vi "Example for Figure Window.vi"() -> ()   [LabVIEW 2020]
panel:
  out "Iteration number":i32
  in  "Stop":bool
  in  "new data":bool
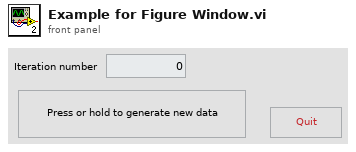
[diagram p1: front panel]
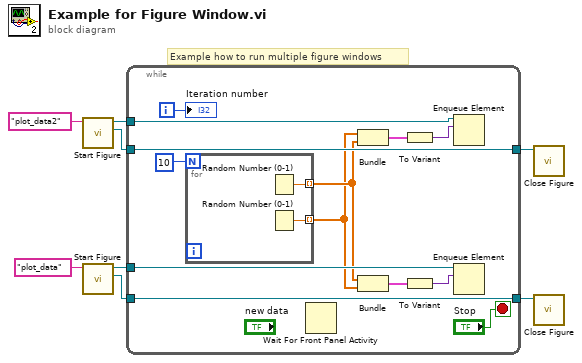
[diagram p0: block diagram]
diagram:
  # "Example how to run multiple figure windows"
  n1 = call "Start Figure.vi"("Qeue name (figure_data)"="plot_data2" ("name (unnamed)")) -> ("reference out"=w4:refnum<vi>, "queue out"=w5:refnum<queue>)  [unwired: 8 in, 1 out]
  n2 = call "Start Figure.vi"("Qeue name (figure_data)"="plot_data" ("name (unnamed)")) -> ("reference out"=w2:refnum<vi>, "queue out"=w6:refnum<queue>)  [unwired: 8 in, 1 out]
  n3 = while {
    tunnel: w6 -> [w20]
    tunnel: [w18] -> w1
    tunnel: w2 -> [w18]
    tunnel: [w17] -> w3
    tunnel: w4 -> [w17]
    tunnel: w5 -> [w16]
    i -> [w19]
    stop <- "Stop" stop-if-true
    n4 = for {
      N: 10 -> [_]
      tunnel: [w23] -> w11 mode=indexing
      tunnel: [w22] -> w10 mode=indexing
      n5 = Random Number (0-1)() -> (number: 0 to 1=w23:dbl)
      n6 = Random Number (0-1)() -> (number: 0 to 1=w22:dbl)
    }
    n7 = Wait For Front Panel Activity() -> ()  [unwired: 3 in, 1 out]
    n8 = Bundle(w10, w11) -> (w9:cluster{dbl[], dbl[]})  [unwired: 1 in]
    n9 = Bundle(w11, w10) -> (w12:cluster{dbl[], dbl[]})  [unwired: 1 in]
    n10 = To Variant(anything=w9) -> (Variant=w13:variant)
    n11 = To Variant(anything=w12) -> (Variant=w14:variant)
    n12 = Enqueue Element(queue=w16, element=w13) -> ()  [unwired: 2 in, 3 out]
    n13 = Enqueue Element(queue=w20, element=w14) -> ()  [unwired: 2 in, 3 out]
    "Iteration number" <- w19
  }
  n14 = call "Close Figure.vi"("reference"=w3) -> ()  [unwired: 10 in, 1 out]
  n15 = call "Close Figure.vi"("reference"=w1) -> ()  [unwired: 10 in, 1 out]
